vi "assert_item_type.vi"(7 "item_type":T1, 8 "error in (no error)":errorcluster, 11 "Item in":refnum<class "Item.lvclass">) -> (0 "error out":errorcluster, 3 "Item out":refnum<class "Item.lvclass">)   [LabVIEW 2020, in "toml_edit.lvlib" / "Item.lvclass"]
uses:
  Item.lvclass
  Item.lvclass/Item.ctl
  type--enum.ctl
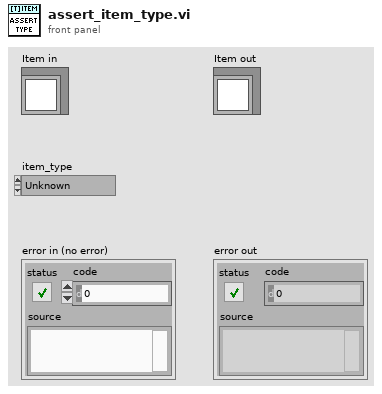
[diagram p1: front panel]
types:
  T1 = typedef "toml_edit.lvlib/Item.lvclass/type--enum.ctl" = enum16{"Unknown", "None", "Value", "ArrayOfTables", "Table"}
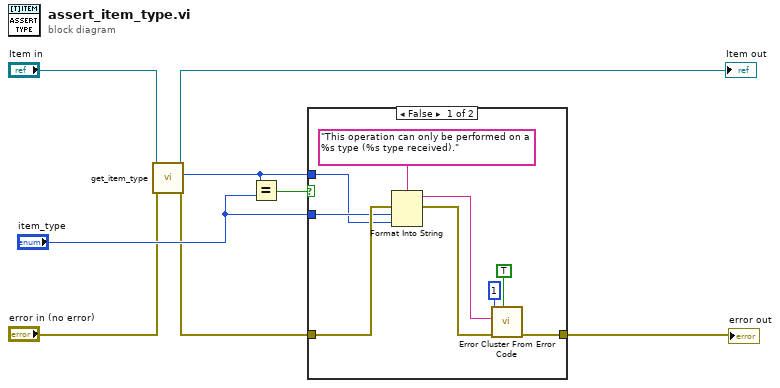
[diagram p0: block diagram]
diagram:
  n1 = call "get_item_type.vi"("error in (no error)"="error in (no error)", "Item in"="Item in") -> ("error out"=w4:errorcluster, "item_type"=w6:T1, "Item out"=→"Item out":refnum<class "Item.lvclass">)  [unwired: 7 in]
  n2 = Equal?(x=w6, y="item_type") -> (x = y?=w5:bool)
  n3 = case shown="False" w5 {
    tunnel: [w14 w18] -> w1
    tunnel: w4 -> [w15 w18]
    tunnel: w6 -> [w9 _]
    tunnel: "item_type" -> [w10 _]
    frame False {
      n4 = Format Into String(format string="This operation can only be performed on a %s type (%s type received).", error in=w15, w10, w9) -> (resulting string=w12:string, error out=w16:errorcluster)  [unwired: 1 in]
      n5 = call <vilib>:"Error Cluster From Error Code.vi"("show call chain? (False)"=TRUE, "error in (no error)"=w16, "error message (\"\")"=w12, "error code (0)"=1) -> ("error out"=w14:errorcluster)  [unwired: 5 in]
    }
    frame True {
    }
  }
  "error out" <- w1
